vi "insert_stack.vi"(9 "novo elemento":T1={"up"=2.0, "down"=1.0}, 10 "pilha input":T1[](array[typedef])) -> (2 "pilha output":T1[](array[typedef]))   [LabVIEW 2016]
uses:
  segment.ctl
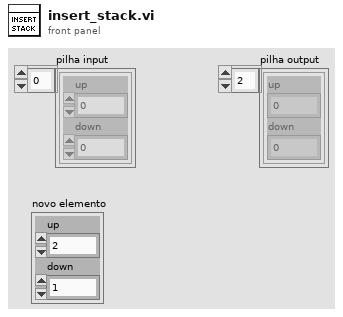
[diagram p1: front panel]
types:
  T1 = typedef "segment.ctl" = cluster{"up":dbl, "down":dbl}
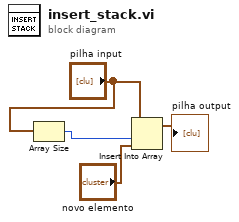
[diagram p0: block diagram]
diagram:
  n1 = Array Size(array="pilha input") -> (size(s)=w1:i32)
  n2 = Insert Into Array(array="pilha input", index=w1, new element="novo elemento") -> (→"pilha output":T1[])
